vi "Format Body.vi"(4 "Indent":string, 6 "Name":string, 7 "Meta Data":string, 8 "Header":string, 9 "Attributes":string, 10 "Body":string, 11 "JSON in":refnum<class "JSON.lvclass">) -> (1 "String out":string, 3 "JSON out":refnum<class "JSON.lvclass">)   [LabVIEW 2019, in "JSON.lvlib" / "JSON.lvclass"]
uses:
  <vilib>/gpm_packages/@cs/persistence/source/JSON/JSON.lvclass
  <vilib>/gpm_packages/@cs/persistence/source/IPersist/IPersist.lvclass
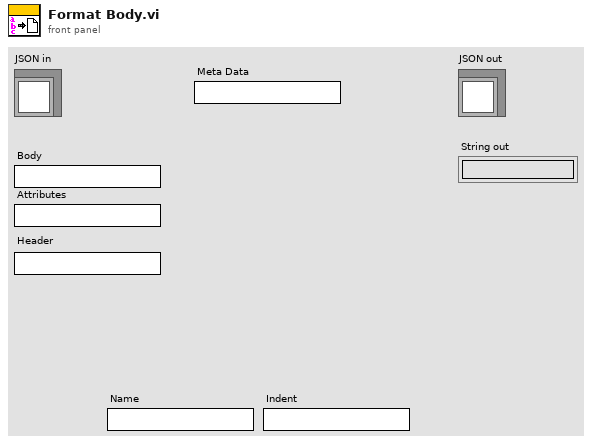
[diagram p1: front panel]
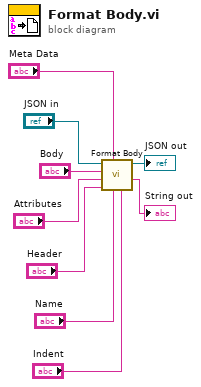
[diagram p0: block diagram]
diagram:
  n1 = call-parent "Format Body.vi"("Indent"="Indent", "Name"="Name", "Meta Data"="Meta Data", "Header"="Header", "Attributes"="Attributes", "Body"="Body", "IPersist in"="JSON in") -> ("String out"=→"String out":string, "IPersist out"=→"JSON out":refnum<class "JSON.lvclass">)  [unwired: 3 in]
